vi "input2sql.vi"() -> ()   [LabVIEW 2015]
uses:
  Controls/STORE_INPUT_NO_CLUSTER.ctl
  Controls/STORE_INPUT_INFORMATION_Cluster.ctl
  <vilib>/addons/database/Connection.llb/DB Tools Open Connec (String).vi
  <vilib>/addons/database/Connection.llb/Conn Execute.vi
  <vilib>/addons/database/Recordset.llb/Rec Destroy - Connection.vi
  <vilib>/addons/database/_DB Variant To Data/Database Variant To Data.xnode
  <vilib>/addons/database/NI_Database_API.lvlib
panel:
  out "Numeric 2":i32
  in  "stop":bool
  out "error out 5":errorcluster
  out "Numeric":i32
  out "error out 4":errorcluster
  out "error out 3":errorcluster
  out "error out 2":errorcluster
  out "error out":errorcluster
  out "Find Array":i32[](array[numeric])
  out "Input No.":string
  out "Table 2":string[][](table)
  out "ECODE":string
  in  "Input Date":timestamp format="%<%d/%m/%Y>T"
  in  "Browse":path=path "\\\\192.168.1.45\\Du Lieu Kho/Data/OutTag" caption="Path"
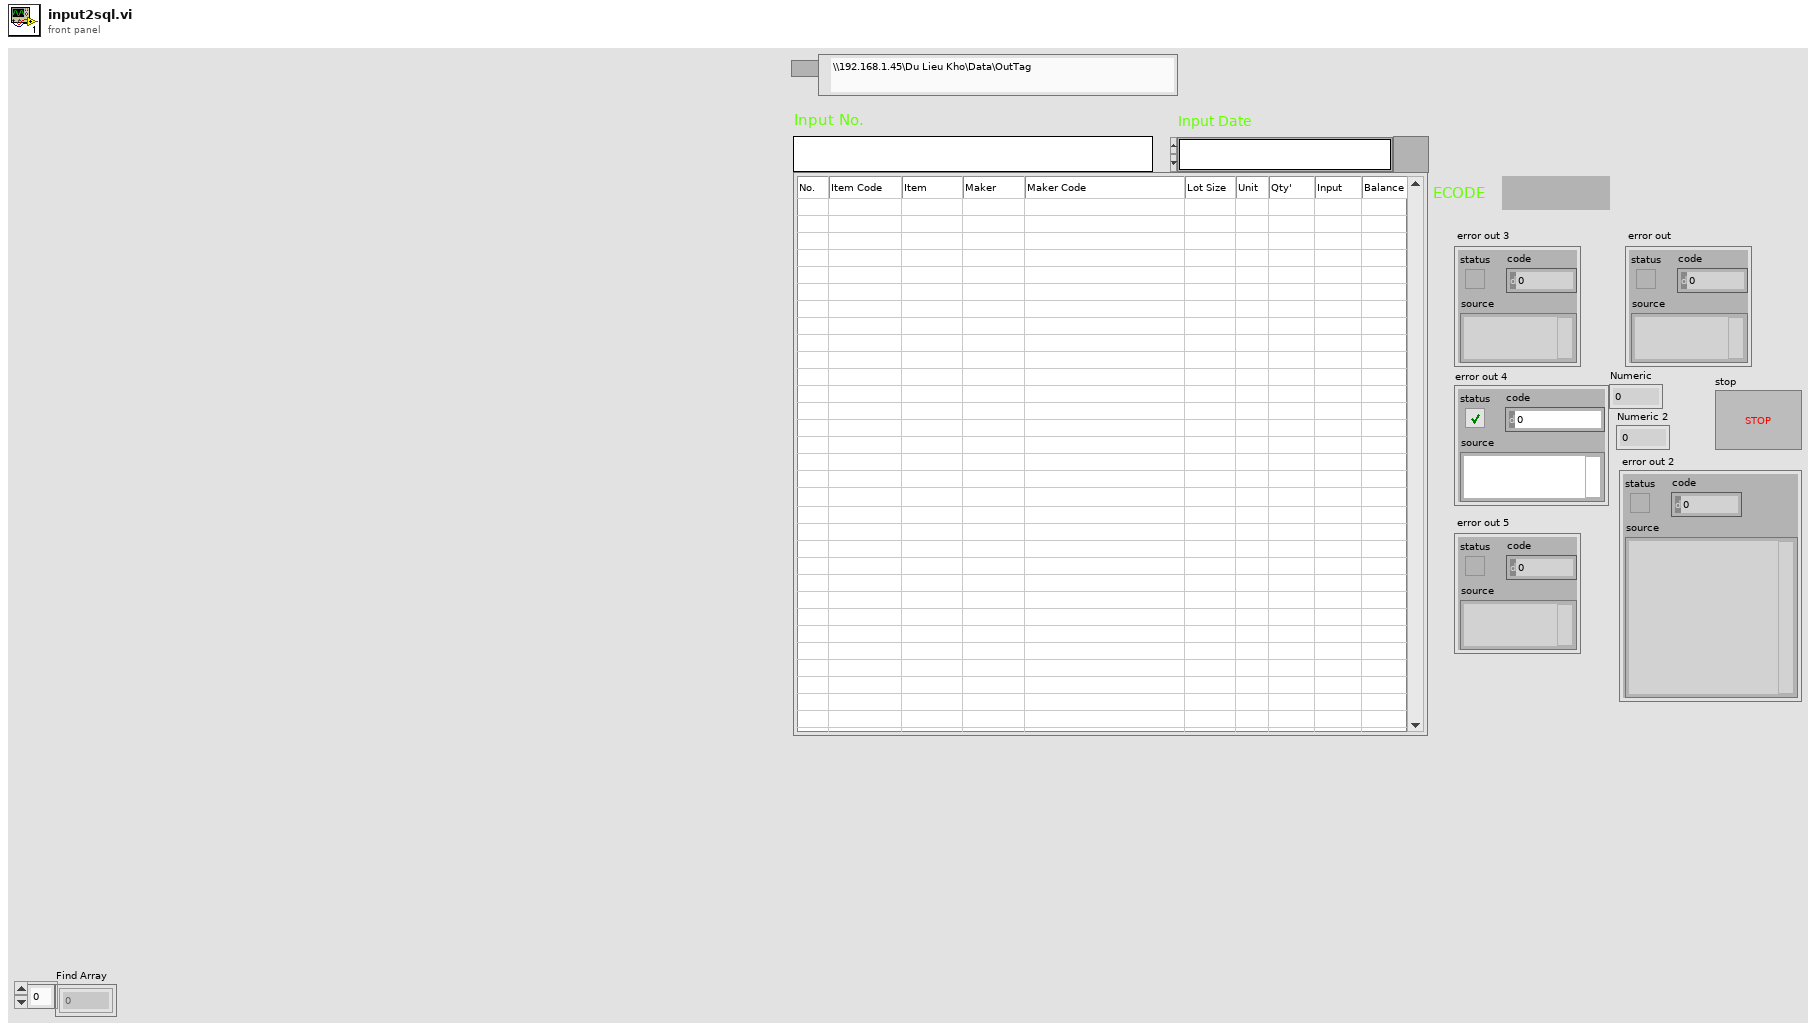
[diagram p1: front panel]
types:
  T1 = typedef "STORE_INPUT_NO_CLUSTER.ctl" = cluster{"NO":dbl, "ITEM_CODE":string, "ITEM":string, "MAKER":string, "MAKER_CODE":string, "LOT_SIZE":dbl, "UNIT":string, "QUANTITY":dbl, "INPUT":dbl, "BALANCE":dbl, "DESTINATION":string, "INVOICE_NO":string}
  T2 = enum16{"open", "replace", "create", "open or create", "replace or create", "replace or create with confirmation"}
  T3 = typedef "STORE_INPUT_INFORMATION_Cluster.ctl" = cluster{"INPUT_NO":string, "INPUT_DATE":timestamp, "ECODE":string}
  T4 = typedef "NI_Database_API.lvlib/Conn ObjectReference.ctl" = refnum<k1>
  T5 = typedef "NI_Database_API.lvlib/Rec ObjectReference.ctl" = refnum<k1>
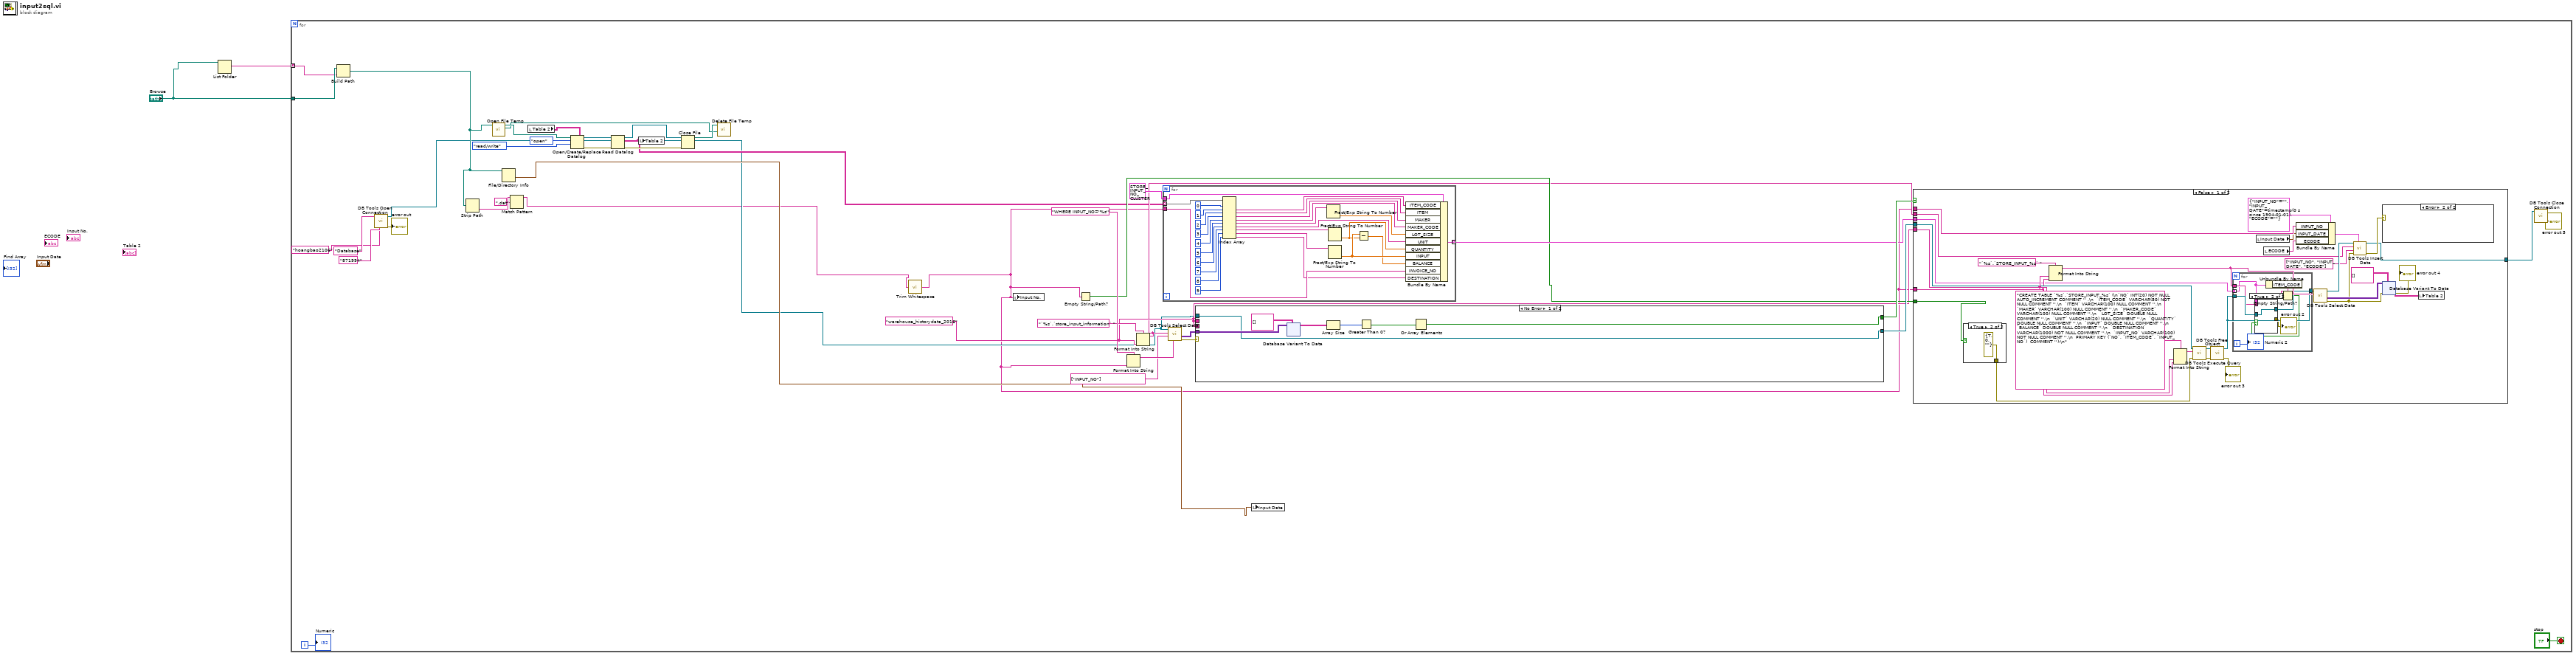
[diagram p0: block diagram]
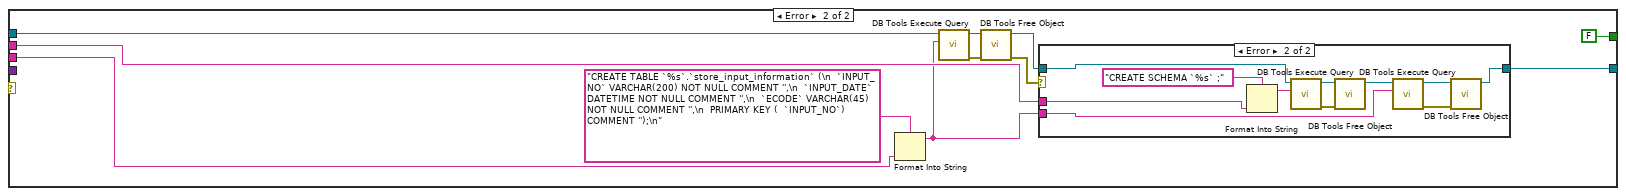
[diagram p2: hidden frame]
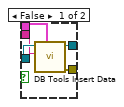
[diagram p6: hidden frame]
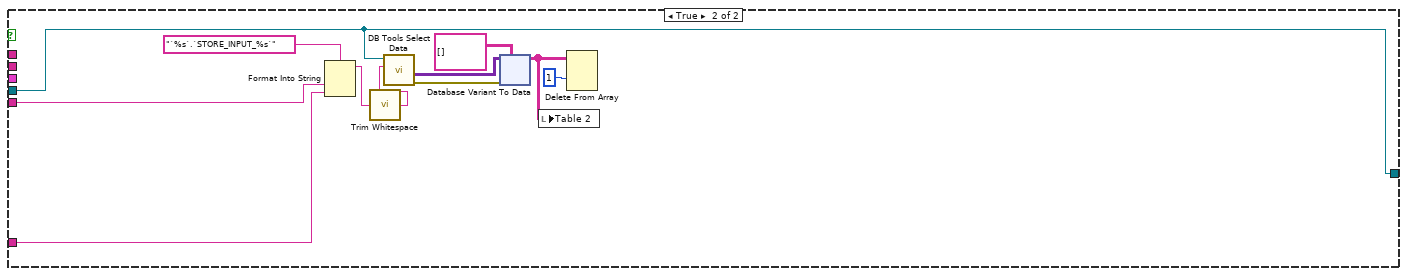
[diagram p7: hidden frame]
diagram:
  n1 = List Folder(path="Browse") -> (filenames=w2:string[])  [unwired: 3 in, 3 out]
  n2 = for {
    tunnel: "Browse" -> [w16]
    tunnel: w2 -> [w15] mode=indexing
    i -> [w13]
    stop <- "stop" stop-if-true
    w22 = "warehouse_historydata_2016"
    n3 = Build Path(base path=w16, name or relative path=w15) -> (appended path=w14:path)
    n4 = call-poly <vilib>:"DB Tools Open Connection.vi"("password"="871994" ("userID"), "userID"="hoangbao2106", "connection information"="Database" ("userID")) -> ("error out"=→"error out":errorcluster, "connection reference"=w8:T4)  [unwired: 5 in]
    n5 = Strip Path(path=w14) -> (name=w19:string)  [unwired: 1 out]
    n6 = call "Open File Temp.vi"("Path file"=w14) -> ("Source Path"=w34:path, "Temp path"=w36:path)  [unwired: 7 in, 2 out]
    n7 = File/Directory Info(path=w14) -> (last mod=w20:timestamp)  [unwired: 1 in, 6 out]
    n8 = Match Pattern(string=w19, regular expression=".dat") -> (before substring=w4:string)  [unwired: 1 in, 3 out]
    n9 = local read "Table 2"() -> (w43:string[][])
    n10 = Open/Create/Replace Datalog(5:w43, 9:enum16{"read/write", "read-only", "write-only"}."read/write" ("access (0:read/write)"), 10:T2."open" ("operation (0:open)"), 11:w36) -> (0:w38:errorcluster, 3:w40:refnum<k1>)  [unwired: 2 in, 1 out]
    n11 = Read Datalog(4:w38, 7:w40) -> (0:w37:errorcluster, 2:w17:string[][], 3:w39:refnum<k1>)  [unwired: 1 in]
    n12 = local write "Table 2"(w17) -> ()
    n13 = Close File(refnum=w39, error in=w37) -> (path=w35:path)  [unwired: 1 out]
    n14 = call "Delete File Temp.vi"("Source Path"=w34, "Temp path"=w35) -> ()  [unwired: 8 in, 2 out]
    n15 = call <vilib>:"Trim Whitespace.vi"("string"=w4) -> ("trimmed string"=w3:string)  [unwired: 1 in]
    n16 = local write "Input No."(w3) -> ()
    n17 = Empty String/Path?(string/path=w3) -> (empty?=w24:bool)
    n18 = Format Into String(format string="WHERE INPUT_NO='%s'", w3) -> (resulting string=w32:string)  [unwired: 2 in, 1 out]
    n19 = Format Into String(format string="`%s`.`store_input_information` ", w22) -> (resulting string=w21:string)  [unwired: 2 in, 1 out]
    n20 = for {
      tunnel: w17 -> [w69] mode=indexing
      tunnel: T1 {"NO"=0.0, "ITEM_CODE"="", "ITEM"="", "MAKER"="", "MAKER_CODE"="", "LOT_SIZE"=0.0, "UNIT"="", "QUANTITY"=0.0, "INPUT"=0.0, "BALANCE"=0.0, "DESTINATION"="", "INVOICE_NO"=""} -> [w70]
      tunnel: [w49] -> w25 mode=indexing
      tunnel: w3 -> [w48]
      n21 = Index Array(array=w69, index #1=0 ("index"), index #2=1 ("index"), index #3=2 ("index"), index #4=3 ("index"), index #5=4 ("index"), index #6=5 ("index"), index #7=6 ("index"), index #8=7 ("index"), index #9=8 ("index"), index #10=9 ("index")) -> (element #2=w58:string, element #3=w57:string, element #4=w56:string, element #5=w55:string, element #6=w54:string, element #7=w52:string, element #8=w51:string, element #9=w50:string, element #10=w44:string)  [unwired: 1 out]
      n22 = Fract/Exp String To Number(string=w54) -> (number=w53:dbl)  [unwired: 3 in, 1 out]
      n23 = Fract/Exp String To Number(string=w51) -> (number=w46:dbl)  [unwired: 3 in, 1 out]
      n24 = Fract/Exp String To Number(string=w50) -> (number=w47:dbl)  [unwired: 3 in, 1 out]
      n25 = Subtract(x=w47, y=w46) -> (x-y=w45:dbl)
      n26 = Bundle By Name(cluster=w70, "ITEM_CODE"=w58, "ITEM"=w57, "MAKER"=w56, "MAKER_CODE"=w55, "LOT_SIZE"=w53, "UNIT"=w52, "QUANTITY"=w46, "INPUT"=w47, "BALANCE"=w45, "INVOICE_NO"=w48, "DESTINATION"=w44) -> (w49:T1)
    }
    n27 = call <vilib>:"DB Tools Select Data.vi"("condition"=w32, "columns"=string[] ["INPUT_NO"], "table"=w21, "connection reference"=w8) -> ("error out"=w28:errorcluster, "data"=w31:variant[][])  [unwired: 2 in, 1 out]
    n28 = case shown="No Error" w28 {
      tunnel: w31 -> [w77 _]
      tunnel: [w72 FALSE] -> w29
      tunnel: w8 -> [w71 w129]
      tunnel: [w71 w125] -> w27
      tunnel: w22 -> [_ w127]
      tunnel: w22 -> [_ w123]
      frame No Error {
        n29 = xnode "Database Variant To Data"("database variant"=w77, "type"=string[][] []) -> ("data"=w75:string[][])  [unwired: 1 in, 1 out]
        n30 = Array Size(array=w75) -> (size(s)=w74:i32[])
        n31 = Greater Than 0?(x=w74) -> (x > 0?=w73:bool[])
        n32 = Or Array Elements(Boolean array=w73) -> (logical OR=w72:bool)
      }
      frame Error {
        n33 = Format Into String(format string="CREATE TABLE `%s`.`store_input_information` (\n  `INPUT_NO` VARCHAR(200) NOT NULL COMMENT '',\n  `INPUT_DATE` DATETIME NOT NULL COMMENT '',\n  `ECODE` VARCHAR(45) NOT NULL COMMENT '',\n  PRIMARY KEY (  `INPUT_NO`)  COMMENT '');\n", w123) -> (resulting string=w122:string)  [unwired: 2 in, 1 out]
        n34 = call-poly <vilib>:"DB Tools Execute Query.vi"("SQL query"=w122, "connection reference"=w129) -> ("error out"=w131:errorcluster, "recordset reference"=w132:T5)  [unwired: 6 in]
        n35 = call-poly <vilib>:"DB Tools Free Object.vi"("error in (no error)"=w131, "recordset reference"=w132) -> ("error out"=w128:errorcluster, "connection reference"=w126:T4)  [unwired: 8 in]
        n36 = case shown="Error" w128 {
          tunnel: w126 -> [w133 w144]
          tunnel: w127 -> [_ w142]
          tunnel: w122 -> [_ w136]
          tunnel: [w133 w135] -> w125
          frame No Error {
          }
          frame Error {
            n37 = Format Into String(format string="CREATE SCHEMA `%s` ;" ("SQL query"), w142) -> (resulting string=w134:string)  [unwired: 2 in, 1 out]
            n38 = call-poly <vilib>:"DB Tools Execute Query.vi"("SQL query"=w134, "connection reference"=w144) -> ("error out"=w140:errorcluster, "recordset reference"=w141:T5)  [unwired: 6 in]
            n39 = call-poly <vilib>:"DB Tools Free Object.vi"("error in (no error)"=w140, "recordset reference"=w141) -> ("connection reference"=w137:T4)  [unwired: 8 in, 1 out]
            n40 = call-poly <vilib>:"DB Tools Execute Query.vi"("SQL query"=w136, "connection reference"=w137) -> ("error out"=w139:errorcluster, "recordset reference"=w138:T5)  [unwired: 6 in]
            n41 = call-poly <vilib>:"DB Tools Free Object.vi"("error in (no error)"=w139, "recordset reference"=w138) -> ("connection reference"=w135:T4)  [unwired: 8 in, 1 out]
          }
        }
      }
    }
    n42 = local write "Input Date"(w20) -> ()
    n43 = case shown="False" w29 {
      tunnel: w27 -> [w173 w243]
      tunnel: w22 -> [w168 w237]
      tunnel: w3 -> [w167 w238]
      tunnel: [w156 w243] -> w7
      tunnel: w25 -> [w166 _]
      tunnel: w21 -> [w159 _]
      tunnel: w3 -> [w155 _]
      tunnel: w24 -> [w149 _]
      frame False {
        n44 = case shown="True" w149 {
          tunnel: [_ errorcluster {"status"=TRUE, "code"=0, "source"=""} ("error constant")] -> w148
          frame False {
          }
          frame True {
          }
        }
        n45 = Format Into String(format string="`%s`.`STORE_INPUT_%s` " ("SQL query"), w168, w167) -> (resulting string=w162:string)  [unwired: 2 in, 1 out]
        n46 = Format Into String(format string="CREATE TABLE `%s`.`STORE_INPUT_%s` (\n`NO` INT(20) NOT NULL AUTO_INCREMENT COMMENT '' ,\n  `ITEM_CODE` VARCHAR(50) NOT NULL COMMENT '',\n  `ITEM` VARCHAR(100) NULL COMMENT '',\n  `MAKER` VARCHAR(100) NULL COMMENT '',\n  `MAKER_CODE` VARCHAR(100) NULL COMMENT '',\n  `LOT_SIZE` DOUBLE NULL COMMENT '',\n  `UNIT` VARCHAR(20) NULL COMMENT '',\n  `QUANTITY` DOUBLE NULL COMMENT '',\n  `INPUT` DOUBLE NULL COMMENT '',\n  `BALANCE` DOUBLE NULL COMMENT '',\n  `DESTINATION` VARCHAR(1000) NOT NULL COMMENT '',\n  `INPUT_NO` VARCHAR(100) NOT NULL COMMENT '',\n  PRIMARY KEY (`NO`, `ITEM_CODE`, `INPUT_NO`)  COMMENT '');\n" ("SQL query"), w168, w167) -> (resulting string=w161:string)  [unwired: 2 in, 1 out]
        n47 = call-poly <vilib>:"DB Tools Execute Query.vi"("error in (no error)"=w148, "SQL query"=w161, "connection reference"=w173) -> ("error out"=w170:errorcluster, "recordset reference"=w171:T5)  [unwired: 5 in]
        n48 = call-poly <vilib>:"DB Tools Free Object.vi"("error in (no error)"=w170, "recordset reference"=w171) -> ("error out"=→"error out 3":errorcluster, "connection reference"=w147:T4)  [unwired: 8 in]
        n49 = for {
          tunnel: w147 -> [w226]
          tunnel: w162 -> [w225]
          tunnel: w166 -> [w222] mode=indexing
          tunnel: [w224] -> _
          i -> [w219]
          n50 = Unbundle By Name(w222) -> ("ITEM_CODE"=w221:string)
          n51 = Empty String/Path?(string/path=w221) -> (empty?=w220:bool)
          n52 = case shown="True" w220 {
            tunnel: w226 -> [w231 w232]
            tunnel: w225 -> [w230 _]
            tunnel: w222 -> [w229 _]
            tunnel: [w228 w232] -> w224
            tunnel: [w227 _] -> w223
            frame False {
              n53 = call <vilib>:"DB Tools Insert Data.vi"("data"=w229, "table"=w230, "connection reference"=w231) -> ("error out"=w227:errorcluster, "connection reference out"=w228:T4)  [unwired: 7 in]
            }
            frame True {
            }
          }
          "error out 2" <- w223
          "Numeric 2" <- w219
        }
        n54 = local read "Input Date"() -> (w154:timestamp)
        n55 = local read "ECODE"() -> (w153:string)
        n56 = Bundle By Name(cluster=T3 {"INPUT_NO"="", "INPUT_DATE"=timestamp(0 s since 1904-01-01), "ECODE"=""} ("INVOICE_INFORMATION_Cluster"), "INPUT_NO"=w155, "INPUT_DATE"=w154, "ECODE"=w153) -> (w152:T3)
        n57 = call <vilib>:"DB Tools Select Data.vi"("table"=w162, "connection reference"=w147) -> ("error out"=w158:errorcluster, "data"=w165:variant[][], "connection reference out"=w160:T4)  [unwired: 4 in]
        n58 = call <vilib>:"DB Tools Insert Data.vi"("data"=w152, "error in (no error)"=w158, "columns"=string[] ["INPUT_NO", "INPUT_DATE", "ECODE"], "table"=w159, "connection reference"=w160) -> ("error out"=w157:errorcluster, "connection reference out"=w156:T4)  [unwired: 5 in]
        n59 = case shown="Error" w157 {
          frame No Error {
          }
          frame Error {
          }
        }
        n60 = xnode "Database Variant To Data"("database variant"=w165, "error in (no error)"=w158, "type"=string[][] []) -> ("data"=w163:string[][], "error out"=→"error out 4":errorcluster)
        n61 = local write "Table 2"(w163) -> ()
      }
      frame True {
        n62 = Format Into String(format string="`%s`.`STORE_INPUT_%s`", w237, w238) -> (resulting string=w234:string)  [unwired: 2 in, 1 out]
        n63 = call <vilib>:"Trim Whitespace.vi"("string"=w234) -> ("trimmed string"=w233:string)  [unwired: 1 in]
        n64 = call <vilib>:"DB Tools Select Data.vi"("table"=w233, "connection reference"=w243) -> ("error out"=w240:errorcluster, "data"=w242:variant[][])  [unwired: 4 in, 1 out]
        n65 = xnode "Database Variant To Data"("database variant"=w242, "error in (no error)"=w240, "type"=string[][] []) -> ("data"=w236:string[][])  [unwired: 1 out]
        n66 = local write "Table 2"(w236) -> ()
        n67 = Delete From Array(array=w236, index (row)=1) -> ()  [unwired: 2 in, 2 out]
      }
    }
    n68 = call <vilib>:"DB Tools Close Connection.vi"("connection reference"=w7) -> ("error out"=→"error out 5":errorcluster)  [unwired: 6 in]
    "Numeric" <- w13
  }
